vi "Bitmap Save As Png.vi"(8 "error in (no error)":errorcluster, 10 "Png Path":path, 11 "Bitmap":refnum<k24>) -> (0 "error out":errorcluster, 3 "Bitmap out":refnum<k24>)   [LabVIEW 2020, in "SvgDotNet.lvlib"]
uses:
  SvgDotNet.lvlib
  System.Drawing
panel:
  # "Connector Pane"
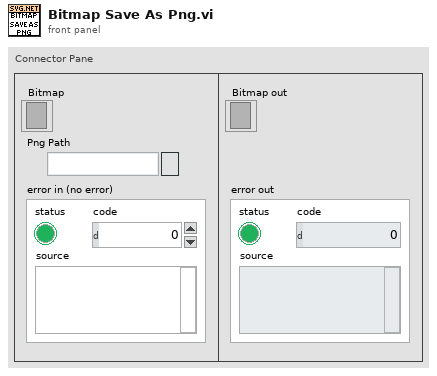
[diagram p1: front panel]
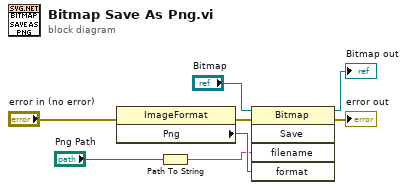
[diagram p0: block diagram]
diagram:
  n1 = property class="ImageFormat"(error in="error in (no error)") -> (error out=w3:errorcluster, "Png"=w8:refnum<k24>)  [unwired: 1 in, 1 out]
  n2 = Path To String(path="Png Path") -> (string=w6:string)
  n3 = invoke class="Bitmap" method="Save"(reference="Bitmap", error in=w3, "filename"=w6, "format"=w8) -> (reference out=→"Bitmap out":refnum<k24>, error out=→"error out":errorcluster)  [unwired: 1 in, 3 out]
